vi "FL_DEC_split_and_filter_for_saving.vi"(2 "Alternative magnets orientation":bool, 3 "Input cluster of SG coefficients":T1, 4 "Filter type":u16(ring)=5 items=["None", "Kalman 0.50", "Kalman 0.30", "Kalman 0.12", "Savitzky-Golay 3/5", "Savitzky-Golay 3/11", "Savitzky-Golay 3/31"], 5 "Offset H.":sgl, 6 "Offset V.":sgl, 7 "DEC input cluster":T3) -> (1 "Magnets coords":T2)   [LabVIEW 2018, in "Tracker.lvlib"]
uses:
  Tracker.lvlib
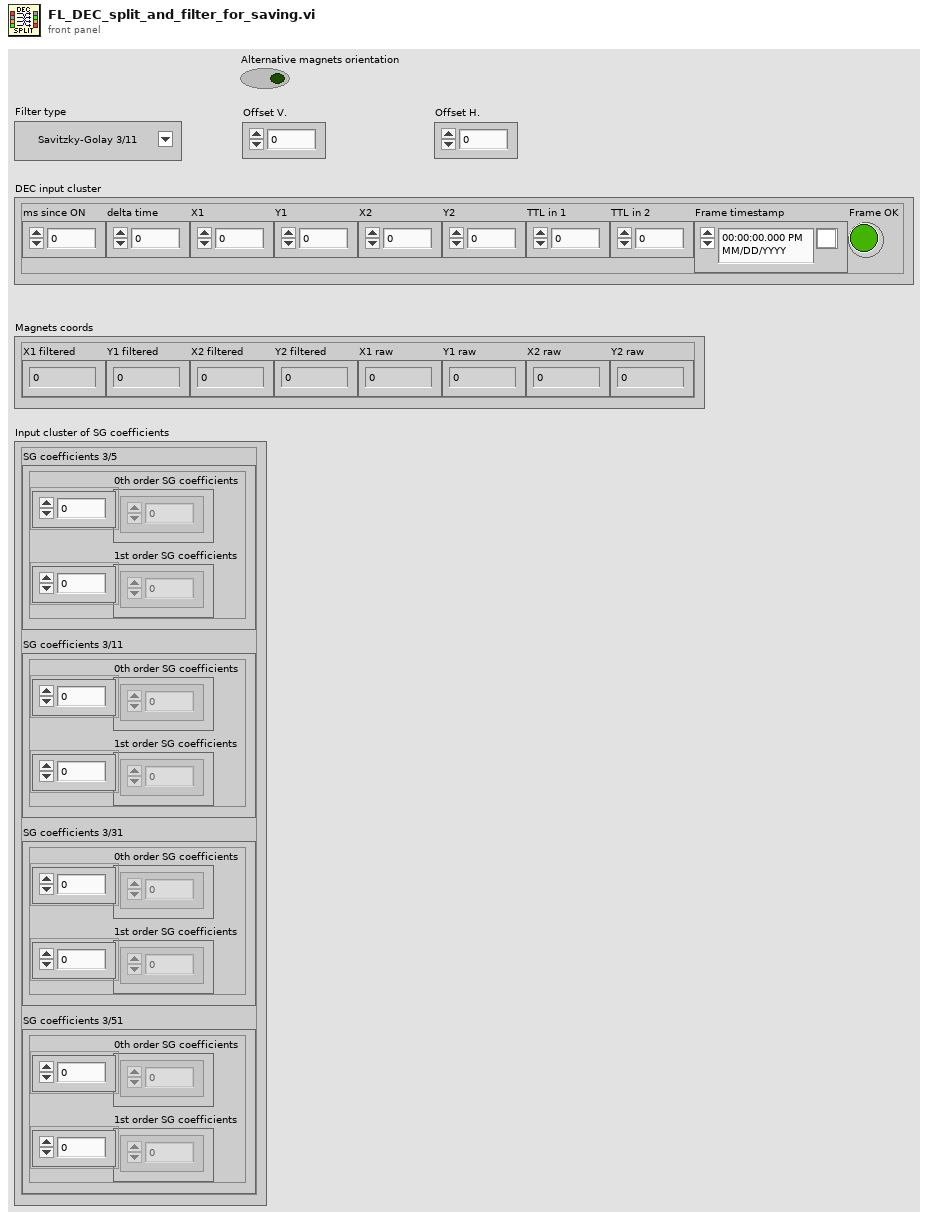
[diagram p1: front panel]
types:
  T1 = cluster{"SG coefficients 3/5":cluster{"0th order SG coefficients":dbl[], "1st order SG coefficients":dbl[]}, "SG coefficients 3/11":cluster{"0th order SG coefficients":dbl[], "1st order SG coefficients":dbl[]}, "SG coefficients 3/31":cluster{"0th order SG coefficients":dbl[], "1st order SG coefficients":dbl[]}, "SG coefficients 3/51":cluster{"0th order SG coefficients":dbl[], "1st order SG coefficients":dbl[]}}
  T2 = cluster{"X1 filtered":dbl, "Y1 filtered":dbl, "X2 filtered":dbl, "Y2 filtered":dbl, "X1 raw":dbl, "Y1 raw":dbl, "X2 raw":dbl, "Y2 raw":dbl}
  T3 = cluster{"ms since ON":u32, "delta time":u32, "X1":sgl, "Y1":sgl, "X2":sgl, "Y2":sgl, "TTL in 1":i16, "TTL in 2":i16, "Frame timestamp":timestamp, "Frame OK":bool}
  T4 = cluster{"X1":dbl, "Y1":dbl, "X2":dbl, "Y2":dbl, sgl, sgl, sgl, sgl}
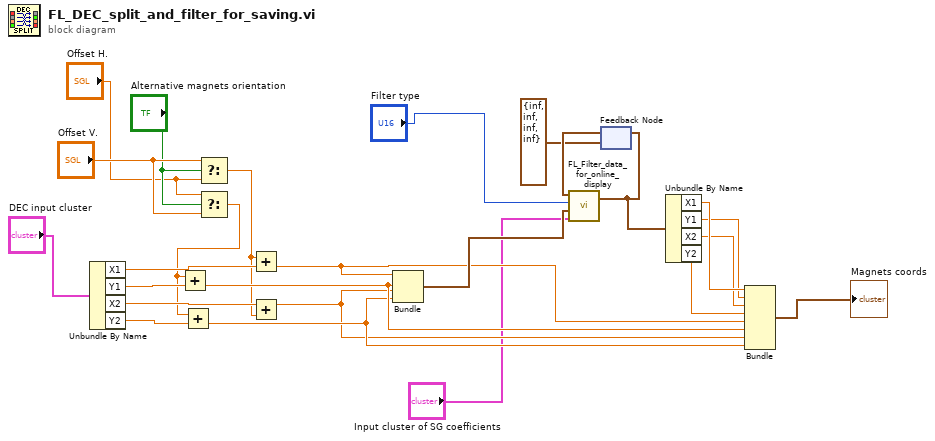
[diagram p0: block diagram]
diagram:
  n1 = Unbundle By Name("DEC input cluster") -> ("X1"=w12:sgl, "Y1"=w15:sgl, "X2"=w11:sgl, "Y2"=w14:sgl)
  n2 = Select(t="Offset V.", s="Alternative magnets orientation", f="Offset H.") -> (s? t:f=w5:sgl)
  n3 = Select(t="Offset H.", s="Alternative magnets orientation", f="Offset V.") -> (s? t:f=w4:sgl)
  n4 = Add(x=w4, y=w15) -> (x+y=w10:sgl)
  n5 = Add(x=w4, y=w14) -> (x+y=w9:sgl)
  n6 = Add(x=w5, y=w12) -> (x+y=w8:sgl)
  n7 = Add(x=w11, y=w5) -> (x+y=w7:sgl)
  n8 = Bundle(w8, w10, w7, w9) -> (w22:cluster{sgl, sgl, sgl, sgl})  [unwired: 1 in]
  n9 = feedback #1(cluster{"X1":dbl, "Y1":dbl, "X2":dbl, "Y2":dbl} {"X1"=inf, "Y1"=inf, "X2"=inf, "Y2"=inf} ("Output data")) -> (w25:cluster{"X1":dbl, "Y1":dbl, "X2":dbl, "Y2":dbl})
  n10 = call "FL_Filter_data_for_online_display.vi"("Input cluster of SG coefficients"="Input cluster of SG coefficients", "Input data"=w22, "Filter type"="Filter type", "Data filtered on previous step"=w25) -> ("Output data"=w21:cluster{"X1":dbl, "Y1":dbl, "X2":dbl, "Y2":dbl})  [unwired: 1 in]
  n11 = feedback-in #1(w21) -> ()
  n12 = Unbundle By Name(w21) -> ("X1"=w19:dbl, "Y1"=w18:dbl, "X2"=w17:dbl, "Y2"=w16:dbl)
  n13 = Bundle("X1"=w19, "Y1"=w18, "X2"=w17, "Y2"=w16, w8, w10, w7, w9) -> (→"Magnets coords":T4)  [unwired: 1 in]
